vi "Example Cluster 3.vi"() -> ()   [LabVIEW 2014]
uses:
  ClusterTypedef1.ctl
  utils/PointerDatatype.lvclass
  utils/PointerInt32Datatype.lvclass
  utils/PointerStringDatatype.lvclass
panel:
  out "Error Out":errorcluster
  in  "Error In":errorcluster
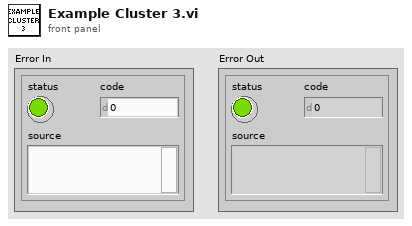
[diagram p1: front panel]
types:
  T1 = typedef "ClusterTypedef1.ctl" = cluster{"some double":dbl}
  T2 = cluster{"NumericConstant inside Cluster":i32, "String Constant inside Cluster":string, "String Array inside Cluster":string[], "String Constant inside Cluster 2":string, dbl, "MyInsideNestedCluster":cluster{"Another Numeric":i32, "some double":dbl, "superNestedCluster":T1}, "myClassName in Cluster":refnum<class "PointerDatatype.lvclass">, "PointerInt32Datatype.lvclass":refnum<class "PointerInt32Datatype.lvclass">, "PointerStringDatatype.lvclass":refnum<class "PointerStringDatatype.lvclass">}
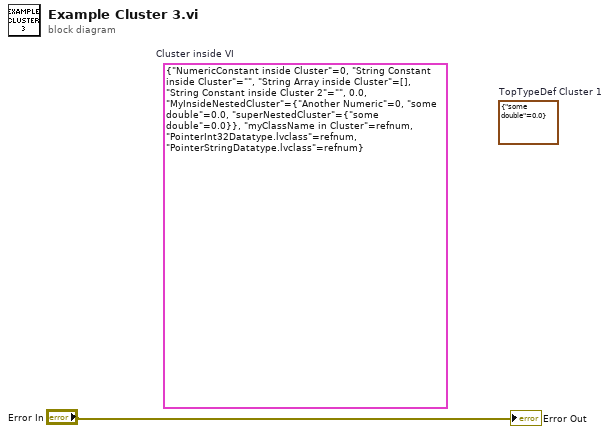
[diagram p0: block diagram]
diagram:
  (unwired) T1 {"some double"=0.0}  # TopTypeDef Cluster 1
  (unwired) T2 {"NumericConstant inside Cluster"=0, "String Constant inside Cluster"="", "String Array inside Cluster"=[], "String Constant inside Cluster 2"="", 0.0, "MyInsideNestedCluster"={"Another Numeric"=0, "some double"=0.0, "superNestedCluster"={"some double"=0.0}}, "myClassName in Cluster"=refnum, "PointerInt32Datatype.lvclass"=refnum, "PointerStringDatatype.lvclass"=refnum}  # Cluster inside VI
  "Error Out" <- "Error In"
